vi "programme principale.vi"() -> ()   [LabVIEW 2019]
uses:
  <vilib>/userDefined/High Color/IMAQdx.ctl
panel:
  in  "Webcam":T1
  out "Déchiffrement":T2(plugin-control)
  out "Chiffrement":T2(plugin-control)
  out "Image Originale":T2(plugin-control)
  out "z":dbl[](array[numeric])
  out "y":dbl[](array[numeric])
  out "x":dbl[](array[numeric])
  # "Projet de Fin d'Etudes\n ISSATSo département de Génie Electronique \nLaboratoire d'Electronique de de Microélectroniqe de la FSM\n    Réalisé par: Soula Achref \nEncadré Par: M. Mohamed GAFSI (Assistant Contractuel à la FSM)"
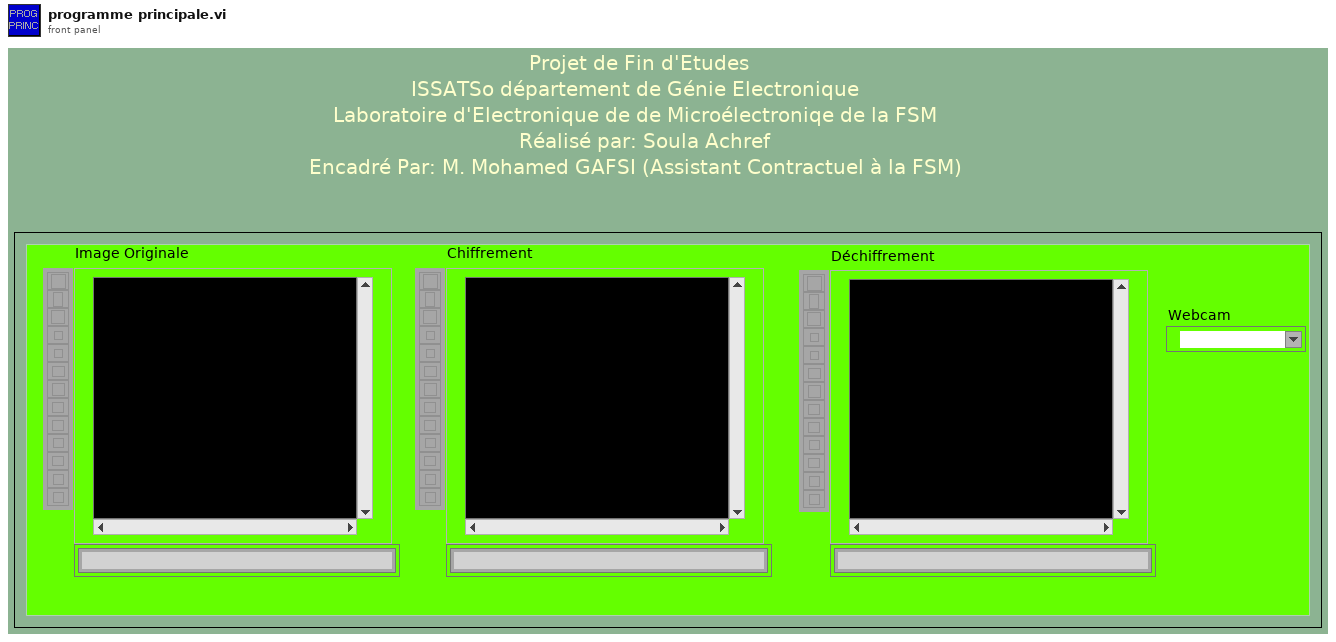
[diagram p1: front panel]
types:
  T1 = typedef "IMAQdx.ctl" = refnum<k21>
  T2 = typedef "IMAQ Image.ctl" = refnum<image>
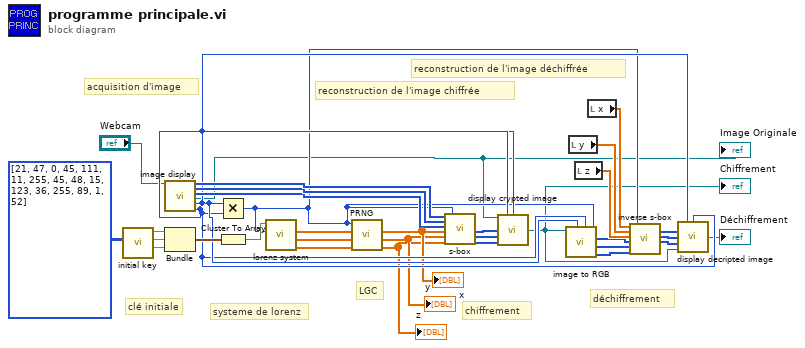
[diagram p0: block diagram]
diagram:
  # "reconstruction de l'image déchiffrée"
  # "reconstruction de l'image chiffrée"
  # "déchiffrement"
  # "chiffrement"
  # "LGC"
  # "acquisition d'image"
  # "systeme de lorenz"
  # "clé initiale"
  n1 = call "initial key.vi"("clé initiale"=u8[][] [[21, 47], [0, 45], [111, 11], [255, 45], [48, 15], [123, 36], [255, 89], [1, 52]]) -> ("Z0"=w32:dbl, "Y0"=w33:dbl, "X0"=w34:dbl)  [unwired: 8 in]
  n2 = call "image display.vi"("webcam"="Webcam") -> ("red out"=w28:u32[], "green out"=w27:u32[], "blue out"=w26:u32[], "original"=w4:T2, "X Resolution"=w22:i32, "Y Resolution"=w21:i32)  [unwired: 13 in]
  "Image Originale" <- w4
  n3 = Bundle("X0"=w34, "Y0"=w33, "Z0"=w32) -> (w31:cluster{"X0":dbl, " Y0":dbl, "Z0":dbl})  [unwired: 1 in]
  n4 = Multiply(x=w22, y=w21) -> (x*y=w8:i32)
  n5 = Cluster To Array(cluster=w31) -> (array=w30:dbl[])
  n6 = call "lorenz system.vi"("Numeric"=w8, "array"=w30) -> ("y"=w12:dbl[], "z"=w13:dbl[], "x"=w14:dbl[])  [unwired: 6 in]
  n7 = call "PRNG.vi"("z"=w12, "y"=w13, "x"=w14, "Numeric"=w8) -> ("z"=w9:dbl[], "y"=w10:dbl[], "x"=w11:dbl[])  [unwired: 5 in]
  "x" <- w11
  "y" <- w10
  "z" <- w9
  n8 = call "s-box.vi"("red in"=w28, "green in"=w27, "blue in"=w26, "x"=w11, "y"=w10, "z"=w9, "Numeric"=w8) -> ("red out"=w17:i32[], "green out"=w16:i32[], "blue out"=w15:i32[])  [unwired: 10 in]
  n9 = call "display crypted image.vi"("image originale"=w4, "X Resolution"=w22, "Y Resolution"=w21, "red in"=w17, "green in"=w16, "blue in"=w15) -> ("image chiffrée"=w2:T2)  [unwired: 9 in]
  "Chiffrement" <- w2
  n10 = call "image to RGB.vi"("Numeric"=w8, "Y Resolution"=w21, "X Resolution"=w22, "image chiffrée"=w2) -> ("blue out"=w18:u32[], "green out"=w19:u32[], "red out"=w20:u32[])  [unwired: 5 in]
  n11 = local read "y"() -> (w24:dbl[])
  n12 = local read "z"() -> (w23:dbl[])
  n13 = local read "x"() -> (w25:dbl[])
  n14 = call "inverse s-box.vi"("x"=w25, "y"=w24, "z"=w23, "red in"=w20, "green in"=w19, "blue in"=w18, "Numeric"=w8) -> ("red out"=w7:u8[], "green out"=w6:u8[], "blue out"=w5:u8[])  [unwired: 10 in]
  n15 = call "display decripted image.vi"("X Resolution"=w22, "Y Resolution"=w21, "red in"=w7, "green in"=w6, "blue in"=w5, "image chiffrée finale"=w2) -> ("image déchiffrée finale"=→"Déchiffrement":T2)  [unwired: 9 in]
